vi "Update Btifle Path.vi"(7 "Bitfile Path Ref":refnum<vi>, 8 "error in (no error)":errorcluster, 11 "Bitfile Path":path) -> (0 "error out":errorcluster)   [LabVIEW 2025, in "I2C Bus Monitor UI.lvlib"]
uses:
  I2C Bus Monitor UI.lvlib
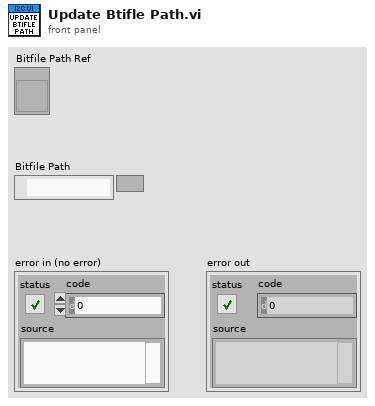
[diagram p1: front panel]
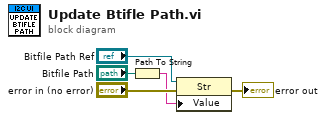
[diagram p0: block diagram]
diagram:
  n1 = Path To String(path="Bitfile Path") -> (string=w3:string)
  n2 = property class="Str"(reference="Bitfile Path Ref", error in="error in (no error)", "Value"=w3) -> (error out=→"error out":errorcluster)  [unwired: 1 out]
